vi "Start and Wait.vi"(8 "error in (no error)":errorcluster, 10 "command (show)":T1=1 items=["show"=1, "hide"=2, "exit"=3]) -> (0 "error out":errorcluster)   [LabVIEW 2009, in "HighFinesse WS5.lvlib"]
doc: "Starts the wavelength meter server and waits until it is done initializing."
uses:
  HighFinesse WS5.lvlib
  Control typedefs.llb/Control Action.ctl
  Private/Wait for Server.vi
  Private/Control.vi
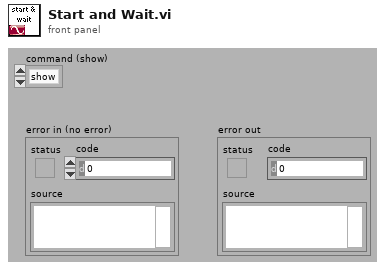
[diagram p1: front panel]
types:
  T1 = typedef "Control Action.ctl" = u32
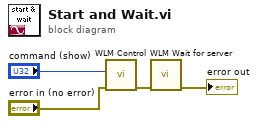
[diagram p0: block diagram]
diagram:
  n1 = call "WLM Control.vi"("error in (no error)"="error in (no error)", "command (show)"="command (show)") -> ("error out"=w4:errorcluster)  [unwired: 9 out]
  n2 = call "WLM Wait for server.vi"("error in (no error)"=w4) -> ("error out"=→"error out":errorcluster)  [unwired: 1 in, 9 out]
